vi "PS采集优化.vi"() -> ()   [LabVIEW 2020]
uses:
  <vilib>/DAQmx/read.llb/DAQmx Read (Counter 1D DBL 1Chan NSamp).vi
  <vilib>/DAQmx/read.llb/DAQmx Read (Counter DBL 1Chan 1Samp).vi
  Global_Variable/Global.vi
  <vilib>/DAQmx/create/channels.llb/DAQmx Create Channel (CI-Period).vi
  <vilib>/DAQmx/configure/timing.llb/DAQmx Timing (Implicit).vi
  <vilib>/DAQmx/miscellaneous.llb/DAQmx Fill In Error Info.vi
  <userlib>/_MGI/1D Array/MGI Average/MGI Average (DBL[]).vi
  <vilib>/DAQmx/create/channels.llb/DAQmx Create Channel (CI-Pulse Width).vi
  <resource>/objmgr/daqmx.rc
panel:
  out "P":dbl
  out "S":dbl
  out "P周期":dbl
  out "S周期":dbl
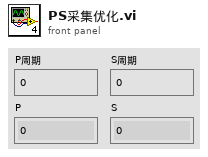
[diagram p1: front panel]
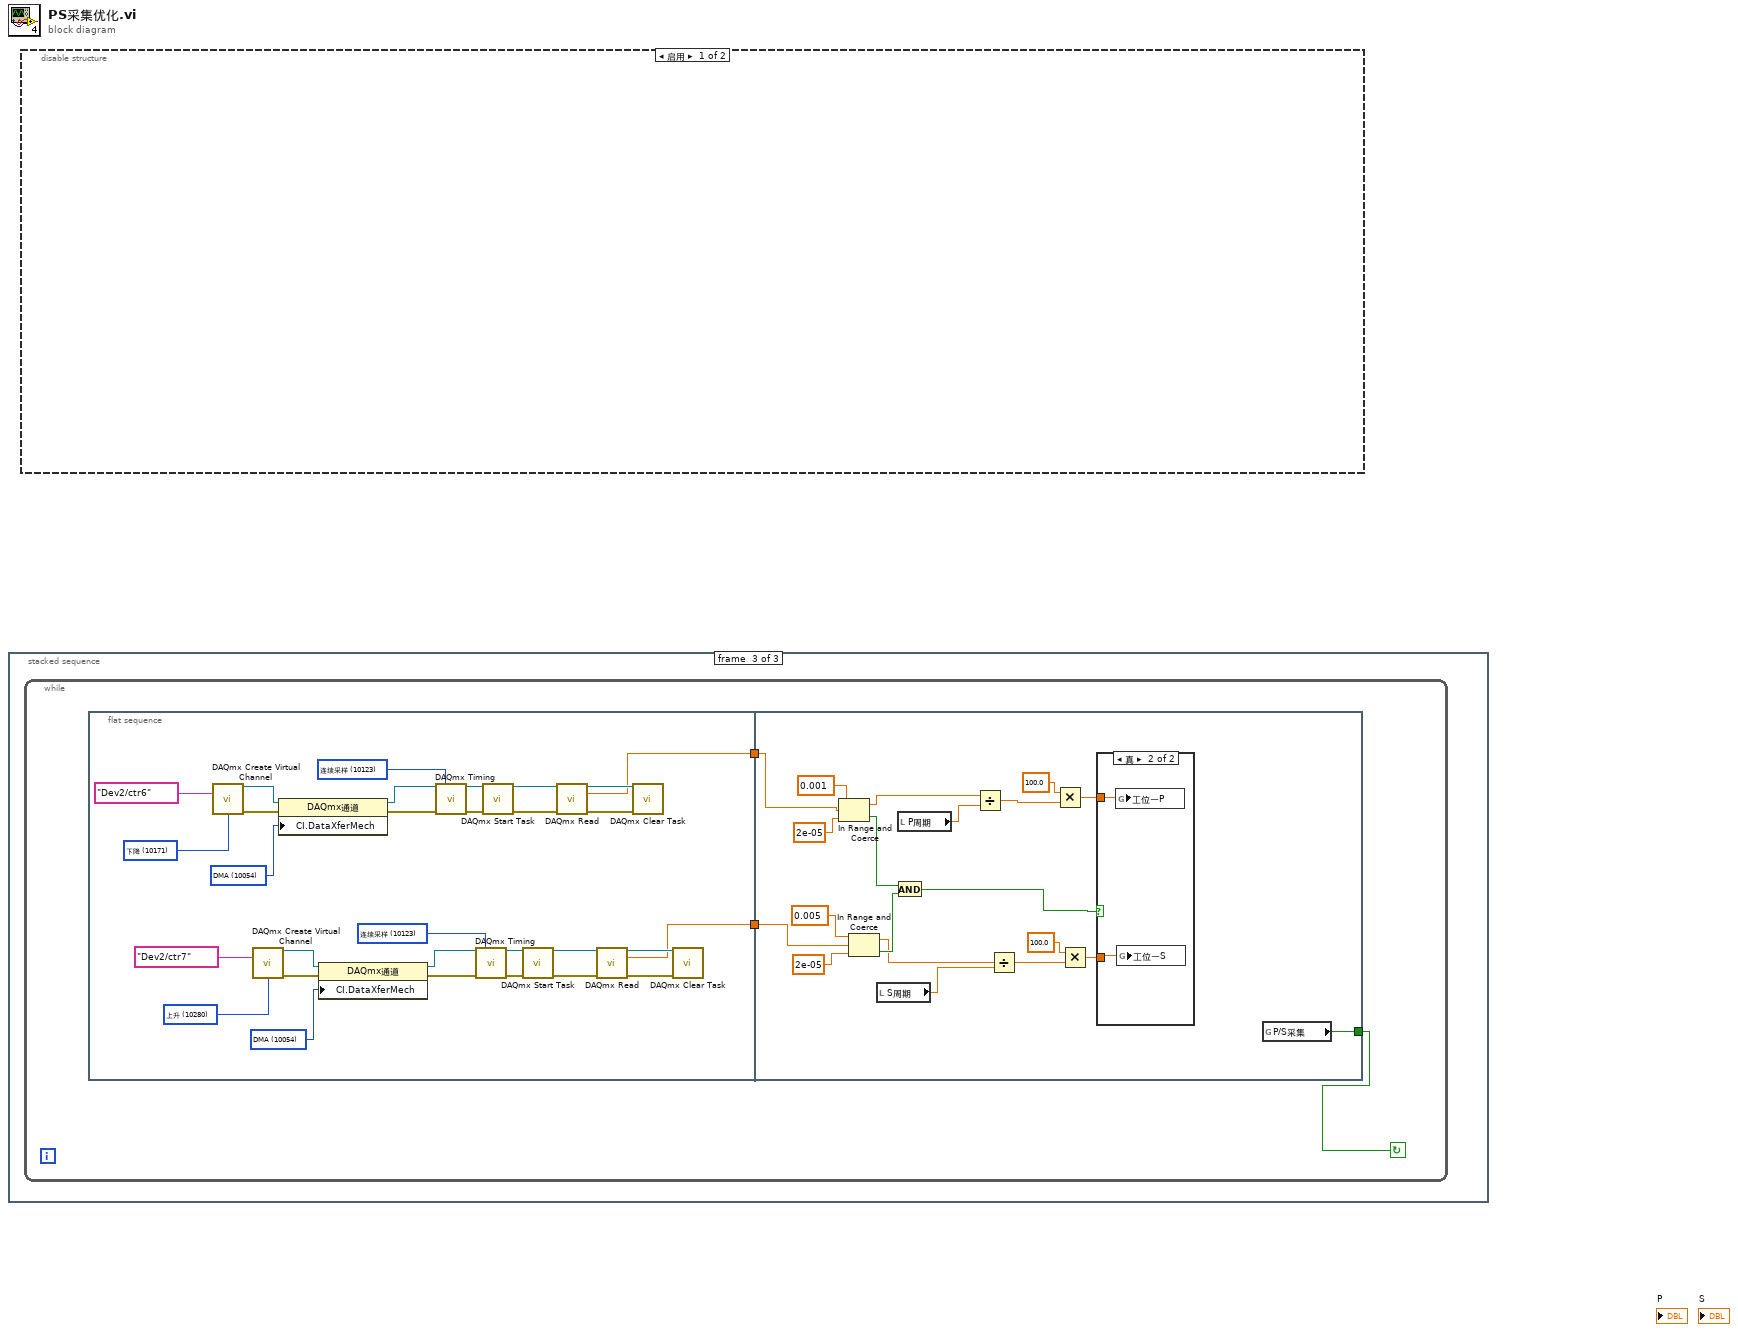
[diagram p0: block diagram]
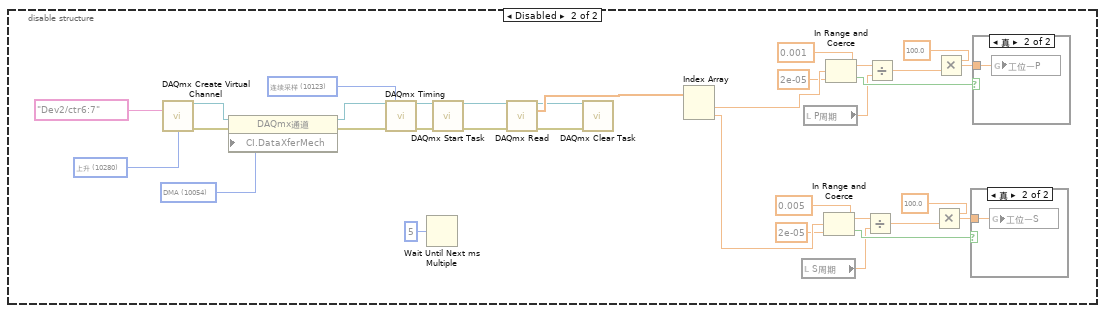
[diagram p2: hidden frame]
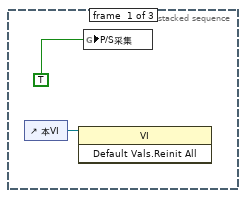
[diagram p5: hidden frame]
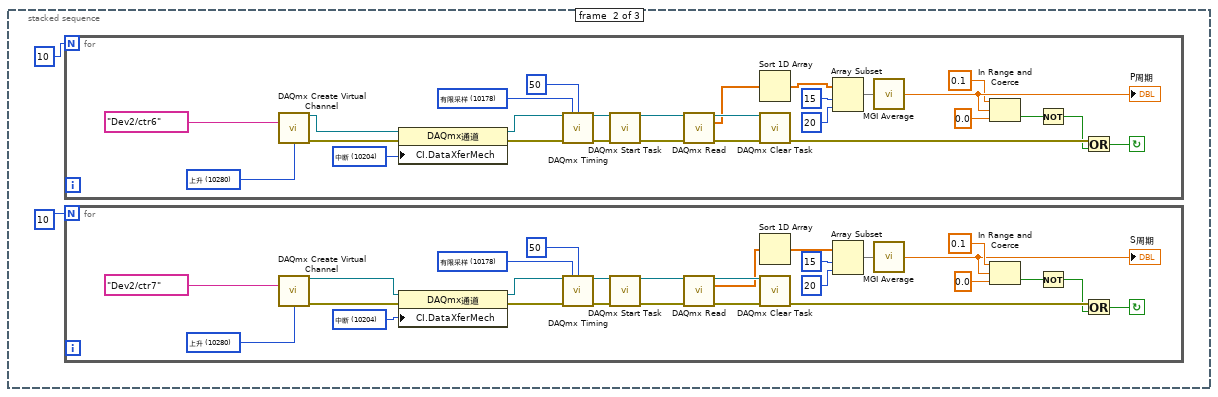
[diagram p6: hidden frame]
diagram:
  n1 = stacked-sequence {
    frame #0 {
      n2 = control-ref of="本VI"() -> (w2:refnum<vi>)
      n3 = invoke class="VI" method="Default Vals.Reinit All"(reference=w2) -> ()  [unwired: 2 in, 3 out]
      n4 = global write "Global.vi" "P/S采集"(TRUE ("工位一占空比采集")) -> ()
    }
    frame #1 {
      n5 = for {
        N: 10 -> [_]
        stop <- w33 continue-if-true
        w45 = 10204 items=["DMA"=10054, "中断"=10204, "程序控制I/O"=10264, "USB Bulk"=12590] ("CI.DataXferMech")
        w49 = 10178 items=["有限采样"=10178, "连续采样"=10123, "硬件定时单点"=12522] ("sample mode")
        w58 = 10280 items=["上升"=10280, "下降"=10171] ("starting edge")
        n6 = call-poly <vilib>:"DAQmx Create Virtual Channel.vi"("counter"=tag "Dev2/ctr6", "starting edge"=w58) -> ("task out"=w57:refnum<k21>, "error out"=w47:errorcluster)  [unwired: 12 in]
        n7 = property class="DAQmx通道"(reference=w57, error in=w47, "CI.DataXferMech"=w45) -> (reference out=w48:refnum<k21>, error out=w46:errorcluster)
        n8 = call-poly <vilib>:"DAQmx Timing.vi"("task/channels in"=w48, "sample mode"=w49, "samples per channel"=50, "error in"=w46) -> ("task out"=w56:refnum<k21>, "error out"=w55:errorcluster)  [unwired: 10 in]
        n9 = call <vilib>:"DAQmx Start Task.vi"("task/channels in"=w56, "error in"=w55) -> ("task out"=w54:refnum<k21>, "error out"=w53:errorcluster)  [unwired: 12 in]
        n10 = call-poly <vilib>:"DAQmx Read.vi"("task/channels in"=w54, "error in"=w53) -> ("task out"=w51:refnum<k21>, "data"=w40:dbl[], "error out"=w52:errorcluster)  [unwired: 11 in]
        n11 = Sort 1D Array(array=w40) -> (sorted array=w43:dbl[])
        n12 = call <vilib>:"DAQmx Clear Task.vi"("task in"=w51, "error in"=w52) -> ("error out"=w35:errorcluster)  [unwired: 13 in]
        n13 = Array Subset(array=w43, index=15 ("索引"), length=20 ("长度")) -> (w32:dbl[])
        n14 = call-poly <userlib>:"MGI Average.vi"("Double[]"=w32) -> ("Average"=w39:dbl)  [unwired: 1 in]
        "P周期" <- w39
        n15 = In Range and Coerce(upper limit=0.1 ("上限"), x=w39, lower limit=0.0 ("上限")) -> (In Range?=w36:bool)  [unwired: 1 out]
        n16 = Not(x=w36) -> (.not. x?=w34:bool)
        n17 = Or(x=w35, y=w34) -> (x .or. y?=w33:bool)
      }
      n18 = for {
        N: 10 -> [_]
        stop <- w6 continue-if-true
        w18 = 10204 items=["DMA"=10054, "中断"=10204, "程序控制I/O"=10264, "USB Bulk"=12590] ("CI.DataXferMech")
        w22 = 10178 items=["有限采样"=10178, "连续采样"=10123, "硬件定时单点"=12522] ("sample mode")
        w31 = 10280 items=["上升"=10280, "下降"=10171] ("starting edge")
        n19 = call-poly <vilib>:"DAQmx Create Virtual Channel.vi"("counter"=tag "Dev2/ctr7", "starting edge"=w31) -> ("task out"=w30:refnum<k21>, "error out"=w20:errorcluster)  [unwired: 12 in]
        n20 = property class="DAQmx通道"(reference=w30, error in=w20, "CI.DataXferMech"=w18) -> (reference out=w21:refnum<k21>, error out=w19:errorcluster)
        n21 = call-poly <vilib>:"DAQmx Timing.vi"("task/channels in"=w21, "sample mode"=w22, "samples per channel"=50, "error in"=w19) -> ("task out"=w29:refnum<k21>, "error out"=w28:errorcluster)  [unwired: 10 in]
        n22 = call <vilib>:"DAQmx Start Task.vi"("task/channels in"=w29, "error in"=w28) -> ("task out"=w27:refnum<k21>, "error out"=w26:errorcluster)  [unwired: 12 in]
        n23 = call-poly <vilib>:"DAQmx Read.vi"("task/channels in"=w27, "error in"=w26) -> ("task out"=w24:refnum<k21>, "data"=w13:dbl[], "error out"=w25:errorcluster)  [unwired: 11 in]
        n24 = Sort 1D Array(array=w13) -> (sorted array=w16:dbl[])
        n25 = call <vilib>:"DAQmx Clear Task.vi"("task in"=w24, "error in"=w25) -> ("error out"=w9:errorcluster)  [unwired: 13 in]
        n26 = Array Subset(array=w16, index=15 ("索引"), length=20 ("长度")) -> (w5:dbl[])
        n27 = call-poly <userlib>:"MGI Average.vi"("Double[]"=w5) -> ("Average"=w10:dbl)  [unwired: 1 in]
        "S周期" <- w10
        n28 = In Range and Coerce(upper limit=0.1 ("上限"), x=w10, lower limit=0.0 ("上限")) -> (In Range?=w8:bool)  [unwired: 1 out]
        n29 = Not(x=w8) -> (.not. x?=w7:bool)
        n30 = Or(x=w9, y=w7) -> (x .or. y?=w6:bool)
      }
    }
    frame #2 {
      n31 = while {
        stop <- w59 continue-if-true
        n32 = flat-sequence {
          tunnel: [w63] -> w61
          tunnel: [w62] -> w60
          tunnel: w61 -> [w93]
          tunnel: w60 -> [w92]
          tunnel: [w94] -> w59
          frame #0 {
            w69 = 10054 items=["DMA"=10054, "中断"=10204, "程序控制I/O"=10264, "USB Bulk"=12590] ("CI.DataXferMech")
            w68 = 10123 items=["有限采样"=10178, "连续采样"=10123, "硬件定时单点"=12522] ("sample mode")
            w67 = 10280 items=["上升"=10280, "下降"=10171] ("starting edge")
            w80 = 10054 items=["DMA"=10054, "中断"=10204, "程序控制I/O"=10264, "USB Bulk"=12590] ("CI.DataXferMech")
            w84 = 10123 items=["有限采样"=10178, "连续采样"=10123, "硬件定时单点"=12522] ("sample mode")
            w91 = 10171 items=["上升"=10280, "下降"=10171] ("starting edge")
            n33 = call-poly <vilib>:"DAQmx Create Virtual Channel.vi"("counter"=tag "Dev2/ctr6", "starting edge"=w91) -> ("task out"=w66:refnum<k21>, "error out"=w82:errorcluster)  [unwired: 12 in]
            n34 = call-poly <vilib>:"DAQmx Create Virtual Channel.vi"("counter"=tag "Dev2/ctr7", "starting edge"=w67) -> ("task out"=w70:refnum<k21>, "error out"=w78:errorcluster)  [unwired: 12 in]
            n35 = property class="DAQmx通道"(reference=w66, error in=w82, "CI.DataXferMech"=w80) -> (reference out=w83:refnum<k21>, error out=w81:errorcluster)
            n36 = property class="DAQmx通道"(reference=w70, error in=w78, "CI.DataXferMech"=w69) -> (reference out=w77:refnum<k21>, error out=w79:errorcluster)
            n37 = call-poly <vilib>:"DAQmx Timing.vi"("task/channels in"=w83, "sample mode"=w84, "error in"=w81) -> ("task out"=w90:refnum<k21>, "error out"=w89:errorcluster)  [unwired: 11 in]
            n38 = call-poly <vilib>:"DAQmx Timing.vi"("task/channels in"=w77, "sample mode"=w68, "error in"=w79) -> ("task out"=w71:refnum<k21>, "error out"=w72:errorcluster)  [unwired: 11 in]
            n39 = call <vilib>:"DAQmx Start Task.vi"("task/channels in"=w90, "error in"=w89) -> ("task out"=w88:refnum<k21>, "error out"=w87:errorcluster)  [unwired: 12 in]
            n40 = call <vilib>:"DAQmx Start Task.vi"("task/channels in"=w71, "error in"=w72) -> ("task out"=w73:refnum<k21>, "error out"=w74:errorcluster)  [unwired: 12 in]
            n41 = call-poly <vilib>:"DAQmx Read.vi"("task/channels in"=w88, "error in"=w87) -> ("task out"=w85:refnum<k21>, "data"=w63:dbl, "error out"=w86:errorcluster)  [unwired: 11 in]
            n42 = call-poly <vilib>:"DAQmx Read.vi"("task/channels in"=w73, "error in"=w74) -> ("task out"=w76:refnum<k21>, "data"=w62:dbl, "error out"=w75:errorcluster)  [unwired: 11 in]
            n43 = call <vilib>:"DAQmx Clear Task.vi"("task in"=w85, "error in"=w86) -> ()  [unwired: 13 in, 1 out]
            n44 = call <vilib>:"DAQmx Clear Task.vi"("task in"=w76, "error in"=w75) -> ()  [unwired: 13 in, 1 out]
          }
          frame #1 {
            n45 = In Range and Coerce(upper limit=0.001 ("上限"), x=w93, lower limit=2e-05 ("下限")) -> (coerced(x)=w105:dbl, In Range?=w109:bool)
            n46 = In Range and Coerce(upper limit=0.005 ("上限"), x=w92, lower limit=2e-05 ("下限")) -> (coerced(x)=w108:dbl, In Range?=w110:bool)
            n47 = local read "S周期"() -> (w107:dbl)
            n48 = And(x=w109, y=w110) -> (x .and. y?=w111:bool)
            n49 = local read "P周期"() -> (w106:dbl)
            n50 = Divide(x=w105, y=w106) -> (x/y=w101:dbl)
            n51 = Divide(x=w108, y=w107) -> (x/y=w102:dbl)
            n52 = Multiply(x=100.0, y=w101) -> (x*y=w104:dbl)
            n53 = Multiply(x=100.0, y=w102) -> (x*y=w103:dbl)
            n54 = case shown="真" w111 {
              tunnel: w103 -> [_ w113]
              tunnel: w104 -> [_ w112]
              frame False {
              }
              frame True {
                n55 = global write "Global.vi" "工位一P"(w112) -> ()
                n56 = global write "Global.vi" "工位一S"(w113) -> ()
              }
            }
            n57 = global read "Global.vi" "P/S采集"() -> (w94:bool)
          }
        }
      }
    }
  }
  n58 = disable-structure shown="启用" {
    frame Enabled {
    }
    frame Disabled {
      w117 = 10054 items=["DMA"=10054, "中断"=10204, "程序控制I/O"=10264, "USB Bulk"=12590] ("CI.DataXferMech")
      w116 = 10123 items=["有限采样"=10178, "连续采样"=10123, "硬件定时单点"=12522] ("sample mode")
      w114 = 10280 items=["上升"=10280, "下降"=10171] ("starting edge")
      n59 = call-poly <vilib>:"DAQmx Create Virtual Channel.vi"("counter"=tag "Dev2/ctr6:7", "starting edge"=w114) -> ("task out"=w134:refnum<k21>, "error out"=w126:errorcluster)  [unwired: 12 in]
      n60 = property class="DAQmx通道"(reference=w134, error in=w126, "CI.DataXferMech"=w117) -> (reference out=w127:refnum<k21>, error out=w125:errorcluster)
      n61 = call-poly <vilib>:"DAQmx Timing.vi"("task/channels in"=w127, "sample mode"=w116, "error in"=w125) -> ("task out"=w133:refnum<k21>, "error out"=w132:errorcluster)  [unwired: 11 in]
      n62 = Wait Until Next ms Multiple(millisecond multiple=u32 5 ("毫秒倍数")) -> ()  [unwired: 1 out]
      n63 = call <vilib>:"DAQmx Start Task.vi"("task/channels in"=w133, "error in"=w132) -> ("task out"=w131:refnum<k21>, "error out"=w130:errorcluster)  [unwired: 12 in]
      n64 = call-poly <vilib>:"DAQmx Read.vi"("task/channels in"=w131, "error in"=w130) -> ("task out"=w128:refnum<k21>, "data"=w135:dbl[], "error out"=w129:errorcluster)  [unwired: 11 in]
      n65 = call <vilib>:"DAQmx Clear Task.vi"("task in"=w128, "error in"=w129) -> ()  [unwired: 13 in, 1 out]
      n66 = Index Array(array=w135) -> (element #1=w143:dbl, element #2=w144:dbl)  [unwired: 2 in]
      n67 = local read "S周期"() -> (w141:dbl)
      n68 = local read "P周期"() -> (w140:dbl)
      n69 = In Range and Coerce(upper limit=0.005 ("上限"), x=w144, lower limit=2e-05 ("下限")) -> (coerced(x)=w142:dbl, In Range?=w147:bool)
      n70 = In Range and Coerce(upper limit=0.001 ("上限"), x=w143, lower limit=2e-05 ("下限")) -> (coerced(x)=w139:dbl, In Range?=w145:bool)
      n71 = Divide(x=w142, y=w141) -> (x/y=w137:dbl)
      n72 = Divide(x=w139, y=w140) -> (x/y=w136:dbl)
      n73 = Multiply(x=100.0, y=w137) -> (x*y=w146:dbl)
      n74 = Multiply(x=100.0, y=w136) -> (x*y=w138:dbl)
      n75 = case shown="真" w147 {
        tunnel: w146 -> [_ w148]
        frame False {
        }
        frame True {
          n76 = global write "Global.vi" "工位一S"(w148) -> ()
        }
      }
      n77 = case shown="真" w145 {
        tunnel: w138 -> [_ w149]
        frame False {
        }
        frame True {
          n78 = global write "Global.vi" "工位一P"(w149) -> ()
        }
      }
    }
  }
